vi "RSD Request Compose.vi"(7 "Checksum used":bool=TRUE, 9 "D-register number":u32=1, 10 "Count number":u8=1, 11 "Address":u8=1) -> (3 "Request":string, 4 "Command":string="RSD")   [LabVIEW 2016, in "Samwontech TEMP2xxx.lvlib"]
uses:
  <instrlib>/Samwontech TEMP2xxx/Samwontech TEMP2xxx.lvlib
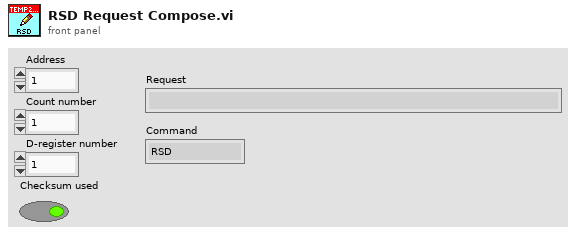
[diagram p1: front panel]
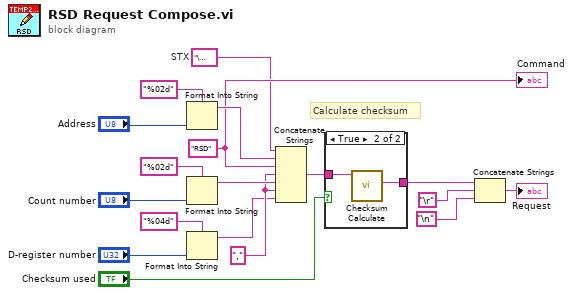
[diagram p0: block diagram]
diagram:
  w14 = "," ("format string")
  w16 = "RSD" ("format string")
  w7 = "\u0002"  # STX
  # "Calculate checksum"
  n1 = Format Into String(format string="%02d", "Address") -> (resulting string=w17:string)  [unwired: 2 in, 1 out]
  n2 = Format Into String(format string="%02d", "Count number") -> (resulting string=w15:string)  [unwired: 2 in, 1 out]
  n3 = Format Into String(format string="%04d", "D-register number") -> (resulting string=w11:string)  [unwired: 2 in, 1 out]
  n4 = Concatenate Strings(w7, w17, w16, w14, w15, w14, w11) -> (w6:string)
  n5 = case shown="True" "Checksum used" {
    tunnel: w6 -> [w19 w21]
    tunnel: [w19 w20] -> w5
    frame False {
    }
    frame True {
      n6 = call <instrlib>:"Checksum Calculate.vi"("Command in"=w21) -> ("Command out (with checksum)"=w20:string)  [unwired: 7 in, 3 out]
    }
  }
  n7 = Concatenate Strings(w5, "\r", "\n") -> (→"Request":string)
  "Command" <- w16
